vi "Grain Boundary Genie, 2014-07-30.vi"() -> ()   [LabVIEW 2010]
uses:
  <vilib>/Analysis/NI_AALBase.lvlib
  <vilib>/Analysis/baseanly.llb/Real Dot Product.vi
  <vilib>/Analysis/NI_AALPro.lvlib
  <vilib>/Analysis/_algsub.llb/Real Vector Norm.vi
  <vilib>/picture/3D Picture Control/NI_3D Picture Control.lvlib
  <vilib>/Analysis/baseanly.llb/A x Vector.vi
  <vilib>/Analysis/baseanly.llb/Vector x A.vi
  <vilib>/Analysis/baseanly.llb/Real A x B.vi
  <vilib>/Utility/file.llb/Write To Spreadsheet File (string).vi
panel:
  out "x/y":dbl[](array[numeric])
  out "Cross Product 2":dbl[](array[numeric])
  out "Cross Product":dbl[](array[numeric])
  out "Lattice Parameter":dbl=6.615785553057252
  in  "Make GB":bool=TRUE
  out "STEM Viewing Angles Array":dbl[][](array[numeric])=[[0.0, 1.0, 0.0], [0.0, 0.0, 1.0], [0.0, 1.0, 1.0], [0.0, -1.0, 1.0], [0.0, 1.0, -1.0]]
  in  "Make Grain 2":bool=TRUE
  in  "Make Grain 1":bool=TRUE
  out "Grain 2 Primative":T1={"Structure Name"="CdTe", "Lattice vector a"=[0.0, 0.0, 6.615785553057252], "Lattice vector b"=[6.615785553057252, 0.0, 0.0], "Lattice vector c"=[0.0, -6.615785553057252, 0.0], "Atoms Array"=[{"Atom Name"="Cd", "Positions (Direct)"=[[0.0, 0.0, 0.0], [0.0, 0.5, 0.5], [0.5, 0.0, 0.5], [0.5, 0.5, 0.0]], "Positions (Cartesian)"=[[0.0, 0.0, 0.0], [3.307892776528626, -3.307892776528626, 0.0], [0.0, -3.307892776528626, 3.307892776528626], [3.307892776528626, 0.0, 3.307892776528626]]}, {"Atom Name"="Te", "Positions (Direct)"=[[0.25, 0.25, 0.25], [0.75, 0.75, 0.25], [0.75, 0.25, 0.75], [0.25, 0.75, 0.75]], "Positions (Cartesian)"=[[1.653946388264313, -1.653946388264313, 1.653946388264313], [4.96183916479294, -1.653946388264313, 4.96183916479294], [1.653946388264313, -4.96183916479294, 4.96183916479294], [4.96183916479294, -4.96183916479294, 1.653946388264313]]}], "# of atoms"=8} {"Atoms Array"."Positions (Cartesian)" format="%#_4f"; "Atoms Array"."Positions (Direct)" format="%#_4f"}
  out "Grain 1 Primitive":T1={"Structure Name"="CdTe", "Lattice vector a"=[0.0, 0.0, 6.615785553057252], "Lattice vector b"=[6.615785553057252, 0.0, 0.0], "Lattice vector c"=[0.0, -6.615785553057252, 0.0], "Atoms Array"=[{"Atom Name"="Cd", "Positions (Direct)"=[[0.0, 0.0, 0.0], [0.0, 0.5, 0.5], [0.5, 0.0, 0.5], [0.5, 0.5, 0.0]], "Positions (Cartesian)"=[[0.0, 0.0, 0.0], [3.307892776528626, -3.307892776528626, 0.0], [0.0, -3.307892776528626, 3.307892776528626], [3.307892776528626, 0.0, 3.307892776528626]]}, {"Atom Name"="Te", "Positions (Direct)"=[[0.25, 0.25, 0.25], [0.75, 0.75, 0.25], [0.75, 0.25, 0.75], [0.25, 0.75, 0.75]], "Positions (Cartesian)"=[[1.653946388264313, -1.653946388264313, 1.653946388264313], [4.96183916479294, -1.653946388264313, 4.96183916479294], [1.653946388264313, -4.96183916479294, 4.96183916479294], [4.96183916479294, -4.96183916479294, 1.653946388264313]]}], "# of atoms"=8} {"Atoms Array"."Positions (Cartesian)" format="%#_4f"; "Atoms Array"."Positions (Direct)" format="%#_4f"}
  in  "Load GB VESTA":bool
  in  "Load G2 VESTA":bool
  in  "Load G1 VESTA":bool
  out "Viewable?":bool=TRUE
  in  "Grain 1 Start":dbl
  in  "Conventional Unit Cell":T1={"Structure Name"="CdTe", "Lattice vector a"=[6.615785553057252, 0.0, 0.0], "Lattice vector b"=[0.0, 6.615785553057252, 0.0], "Lattice vector c"=[0.0, 0.0, 6.615785553057252], "Atoms Array"=[{"Atom Name"="Cd", "Positions (Direct)"=[[0.0, 0.0, 0.0], [0.0, 0.5, 0.5], [0.5, 0.0, 0.5], [0.5, 0.5, 0.0]], "Positions (Cartesian)"=[[0.0, 0.0, 0.0], [0.0, 3.307892776528626, 3.307892776528626], [3.307892776528626, 0.0, 3.307892776528626], [3.307892776528626, 3.307892776528626, 0.0]]}, {"Atom Name"="Te", "Positions (Direct)"=[[0.25, 0.25, 0.25], [0.75, 0.75, 0.25], [0.75, 0.25, 0.75], [0.25, 0.75, 0.75]], "Positions (Cartesian)"=[[1.653946388264313, 1.653946388264313, 1.653946388264313], [4.96183916479294, 4.96183916479294, 1.653946388264313], [4.96183916479294, 1.653946388264313, 4.96183916479294], [1.653946388264313, 4.96183916479294, 4.96183916479294]]}], "# of atoms"=8}
  in  "Overlap Region":dbl(slide) scale=-2.0..2.0
  in  "Tab Control":T2(tab)=enum."Analysis"
  in  "Remove Close Atoms":bool
  out "Subset for Y?":bool
  out "Repeating Y Length Scale":dbl=99.01964045547014
  in  "Crop to Smallest Repeating":bool
  in  "Slab Y":dbl=6.0
  in  "Slab X":dbl=6.0
  out "Subset for X?":bool
  in  "Tolerance (A)":dbl=1.0
  in  "Presorted?":bool
  out "Repeating X Length Scale":dbl=99.01964045547014
  in  "Minimally Allowable Distance (A)":dbl=1.5
  out "# of Atoms Removed":i32
  in  "Options":cluster{"Border?":bool, "Bonds?":bool}={"Border?"=TRUE, "Bonds?"=FALSE}
  in  "Scale":dbl(slide)=0.06161137440758294 scale=0.0..0.2
  in  "Mutual Viewing Angle":dbl[](array[numeric])=[0.0, 1.0, 0.0]
  in  "STEM Viewing Angles":u16(ring) items=["[0,0,1]", "[1,-1,0]", "[-1,1,0]"]
  out "# of Atoms":i32=36
  out "Atoms / A³":dbl=0.06216246776245014
  out "% of Bulk atomic density":dbl=2.250005167366452
  out "Grain 2 Integers":dbl[](array[numeric])=[1.0, 0.0, 0.0]
  out "Grain 1 Integers":dbl[](array[numeric])=[1.0, 0.0, 0.0]
  out "Misorientation Angle":dbl
  out "Suggested Viewing Angle":dbl[](array[numeric])=[0.0, 1.0, 0.0]
  in  "Suggest Sizes":bool
  in  "Tolerance":dbl=0.01
  in  "Grain 2 Max Length (A)":dbl=10.0
  in  "Grain 1 Max Length (A)":dbl=10.0
  in  "Max Grain Width":dbl=1.0
  in  "Grain 2 Min Length":dbl=1.0
  in  "Grain 1 Min Length (A)":dbl=1.0
  in  "Max Grain Height":dbl=1.0
  in  "Structure Name":string="(0.0) twist [1,0,0] [1,0,0+0.0tilt] (0.00,0.00,0.00)T GB"
  in  "Save to POSCAR":bool
  in  "Relaxation Type":string(combo)="conv opti"
  in  "Make into GULP":bool
  out "Grain Boundary Object":refnum<vi>
  out "Grain 2 Object":refnum<vi>
  out "Grain 1 Object":refnum<vi>
  in  "Add Tilt Angle":dbl(slide) scale=0.0..90.0
  out "Grain Boundary":T1={"Structure Name"="(0.0) twist [1,0,0] [1,0,0+0.0tilt] (0.00,0.00,0.00)T GB", "Lattice vector a"=[6.615785553057252, 0.0, 0.0], "Lattice vector b"=[0.0, 6.615785553057252, 0.0], "Lattice vector c"=[0.0, 0.0, 13.231571106114504], "Atoms Array"=[{"Atom Name"="Cd", "Positions (Direct)"=[[0.0, 0.0, 0.0], [0.0, 0.0, 0.5], [0.0, 0.5, 0.25], [0.0, 1.0, 0.0], [0.0, 1.0, 0.5], [0.5, 0.0, 0.25], [0.5, 0.5, 0.0], [0.5, 0.5, 0.5], [0.5, 1.0, 0.25], [1.0, 0.0, 0.0], [1.0, 0.0, 0.5], [1.0, 0.5, 0.25], [1.0, 1.0, 0.0], [1.0, 1.0, 0.5], [0.0, 0.0, 0.5], [0.0, 0.0, 1.0], [0.0, 0.5, 0.75], [0.0, 1.0, 0.5], [0.0, 1.0, 1.0], [0.5, 0.0, 0.75], [0.5, 0.5, 0.5], [0.5, 0.5, 1.0], [0.5, 1.0, 0.75], [1.0, 0.0, 0.5], [1.0, 0.0, 1.0], [1.0, 0.5, 0.75], [1.0, 1.0, 0.5], [1.0, 1.0, 1.0]], "Positions (Cartesian)"=[[0.0, 0.0, 0.0], [0.0, 0.0, 6.615785553057252], [0.0, 3.307892776528626, 3.307892776528626], [0.0, 6.615785553057252, 0.0], [0.0, 6.615785553057252, 6.615785553057252], [3.307892776528626, 0.0, 3.307892776528626], [3.307892776528626, 3.307892776528626, 0.0], [3.307892776528626, 3.307892776528626, 6.615785553057252], [3.307892776528626, 6.615785553057252, 3.307892776528626], [6.615785553057252, 0.0, 0.0], [6.615785553057252, 0.0, 6.615785553057252], [6.615785553057252, 3.307892776528626, 3.307892776528626], [6.615785553057252, 6.615785553057252, 0.0], [6.615785553057252, 6.615785553057252, 6.615785553057252], [0.0, 0.0, 6.615785553057252], [0.0, 0.0, 13.231571106114504], [0.0, 3.307892776528626, 9.92367832958588], [0.0, 6.615785553057252, 6.615785553057252], [0.0, 6.615785553057252, 13.231571106114504], [3.307892776528626, 0.0, 9.92367832958588], [3.307892776528626, 3.307892776528626, 6.615785553057252], [3.307892776528626, 3.307892776528626, 13.231571106114504], [3.307892776528626, 6.615785553057252, 9.92367832958588], [6.615785553057252, 0.0, 6.615785553057252], [6.615785553057252, 0.0, 13.231571106114504], [6.615785553057252, 3.307892776528626, 9.92367832958588], [6.615785553057252, 6.615785553057252, 6.615785553057252], [6.615785553057252, 6.615785553057252, 13.231571106114504]]}, {"Atom Name"="Te", "Positions (Direct)"=[[0.25, 0.24999999999999992, 0.375], [0.25, 0.75, 0.125], [0.75, 0.24999999999999992, 0.125], [0.75, 0.75, 0.375], [0.25, 0.24999999999999992, 0.875], [0.25, 0.75, 0.625], [0.75, 0.24999999999999992, 0.625], [0.75, 0.75, 0.875]], "Positions (Cartesian)"=[[1.653946388264313, 1.6539463882643126, 4.96183916479294], [1.653946388264313, 4.96183916479294, 1.653946388264313], [4.96183916479294, 1.6539463882643126, 1.653946388264313], [4.96183916479294, 4.96183916479294, 4.96183916479294], [1.653946388264313, 1.6539463882643126, 11.577624717850192], [1.653946388264313, 4.96183916479294, 8.269731941321565], [4.96183916479294, 1.6539463882643126, 8.269731941321565], [4.96183916479294, 4.96183916479294, 11.577624717850192]]}], "# of atoms"=36} {"Atoms Array"."Positions (Cartesian)" format="%#_4f"; "Atoms Array"."Positions (Direct)" format="%#_4f"}
  out "Grain 2":T1={"Structure Name"="CdTe Expanded to Box", "Lattice vector a"=[6.615785553057252, 0.0, 0.0], "Lattice vector b"=[0.0, 6.615785553057252, 0.0], "Lattice vector c"=[0.0, 0.0, 6.615785553057252], "Atoms Array"=[{"Atom Name"="Cd", "Positions (Direct)"=[[0.0, 0.0, 0.0], [0.0, 0.0, 1.0], [0.0, 0.5, 0.5], [0.0, 1.0, 0.0], [0.0, 1.0, 1.0], [0.5, 0.0, 0.5], [0.5, 0.5, 0.0], [0.5, 0.5, 1.0], [0.5, 1.0, 0.5], [1.0, 0.0, 0.0], [1.0, 0.0, 1.0], [1.0, 0.5, 0.5], [1.0, 1.0, 0.0], [1.0, 1.0, 1.0]], "Positions (Cartesian)"=[[0.0, 0.0, 0.0], [0.0, 0.0, 6.615785553057252], [0.0, 3.307892776528626, 3.307892776528626], [0.0, 6.615785553057252, 0.0], [0.0, 6.615785553057252, 6.615785553057252], [3.307892776528626, 0.0, 3.307892776528626], [3.307892776528626, 3.307892776528626, 0.0], [3.307892776528626, 3.307892776528626, 6.615785553057252], [3.307892776528626, 6.615785553057252, 3.307892776528626], [6.615785553057252, 0.0, 0.0], [6.615785553057252, 0.0, 6.615785553057252], [6.615785553057252, 3.307892776528626, 3.307892776528626], [6.615785553057252, 6.615785553057252, 0.0], [6.615785553057252, 6.615785553057252, 6.615785553057252]]}, {"Atom Name"="Te", "Positions (Direct)"=[[0.25, 0.24999999999999992, 0.75], [0.25, 0.75, 0.25], [0.75, 0.24999999999999992, 0.25], [0.75, 0.75, 0.75]], "Positions (Cartesian)"=[[1.653946388264313, 1.6539463882643126, 4.96183916479294], [1.653946388264313, 4.96183916479294, 1.653946388264313], [4.96183916479294, 1.6539463882643126, 1.653946388264313], [4.96183916479294, 4.96183916479294, 4.96183916479294]]}], "# of atoms"=18} {"Atoms Array"."Positions (Cartesian)" format="%#_4f"; "Atoms Array"."Positions (Direct)" format="%#_4f"}
  out "Grain 1":T1={"Structure Name"="CdTe Expanded to Box", "Lattice vector a"=[6.681943408587824, 0.0, 0.0], "Lattice vector b"=[0.0, 6.681943408587824, 0.0], "Lattice vector c"=[0.0, 0.0, 6.615785553057252], "Atoms Array"=[{"Atom Name"="Cd", "Positions (Direct)"=[[0.0, 0.0, 0.0], [0.0, 0.0, 1.0], [0.0, 0.49504950495049505, 0.5], [0.0, 0.9900990099009901, 0.0], [0.0, 0.9900990099009901, 1.0], [0.49504950495049505, 0.0, 0.5], [0.49504950495049505, 0.49504950495049505, 0.0], [0.49504950495049505, 0.49504950495049505, 1.0], [0.49504950495049505, 0.9900990099009901, 0.5], [0.9900990099009901, 0.0, 0.0], [0.9900990099009901, 0.0, 1.0], [0.9900990099009901, 0.49504950495049505, 0.5], [0.9900990099009901, 0.9900990099009901, 0.0], [0.9900990099009901, 0.9900990099009901, 1.0]], "Positions (Cartesian)"=[[0.0, 0.0, 0.0], [0.0, 0.0, 6.615785553057252], [0.0, 3.307892776528626, 3.307892776528626], [0.0, 6.615785553057252, 0.0], [0.0, 6.615785553057252, 6.615785553057252], [3.307892776528626, 0.0, 3.307892776528626], [3.307892776528626, 3.307892776528626, 0.0], [3.307892776528626, 3.307892776528626, 6.615785553057252], [3.307892776528626, 6.615785553057252, 3.307892776528626], [6.615785553057252, 0.0, 0.0], [6.615785553057252, 0.0, 6.615785553057252], [6.615785553057252, 3.307892776528626, 3.307892776528626], [6.615785553057252, 6.615785553057252, 0.0], [6.615785553057252, 6.615785553057252, 6.615785553057252]]}, {"Atom Name"="Te", "Positions (Direct)"=[[0.24752475247524752, 0.24752475247524747, 0.75], [0.24752475247524752, 0.7425742574257427, 0.25], [0.7425742574257427, 0.24752475247524747, 0.25], [0.7425742574257427, 0.7425742574257427, 0.75]], "Positions (Cartesian)"=[[1.653946388264313, 1.6539463882643126, 4.96183916479294], [1.653946388264313, 4.96183916479294, 1.653946388264313], [4.96183916479294, 1.6539463882643126, 1.653946388264313], [4.96183916479294, 4.96183916479294, 4.96183916479294]]}], "# of atoms"=18} {"Atoms Array"."Positions (Cartesian)" format="%#_4f"; "Atoms Array"."Positions (Direct)" format="%#_4f"}
  in  "Primitive Lattice Vectors":T1={"Structure Name"="Relax2 Subcrystal", "Lattice vector a"=[0.0, 3.3046962263585, 3.3046962263585], "Lattice vector b"=[3.3046962263585, 0.0, 3.3046962263585], "Lattice vector c"=[3.3046962263585, 3.3046962263585, 0.0], "Atoms Array"=[{"Atom Name"="Cd", "Positions (Direct)"=[[0.0, 0.0, 0.0]], "Positions (Cartesian)"=[[0.0, 0.0, 0.0]]}, {"Atom Name"="Te", "Positions (Direct)"=[[0.25, 0.25, 0.25]], "Positions (Cartesian)"=[[1.65234811317925, 1.65234811317925, 1.65234811317925]]}], "# of atoms"=2} {"Atoms Array"."Positions (Cartesian)" format="%#_4f"; "Atoms Array"."Positions (Direct)" format="%#_4f"}
  out "Grain Boundary Render":refnum<vi>(3d-picture)
  in  "Translation Vector":dbl[](array[slide])=[0.0, 0.0, 0.0] scale=0.0..2.0
  in  "Twist Angle":dbl(slide) scale=0.0..90.0
  in  "Grain 2 Orientation":dbl[](array[numeric])=[1.0, 0.0, 0.0]
  in  "Grain 1 Orientation":dbl[](array[numeric])=[1.0, 0.0, 0.0]
  out "Grain 2 Render":refnum<vi>(3d-picture)
  out "Grain 1 Render":refnum<vi>(3d-picture)
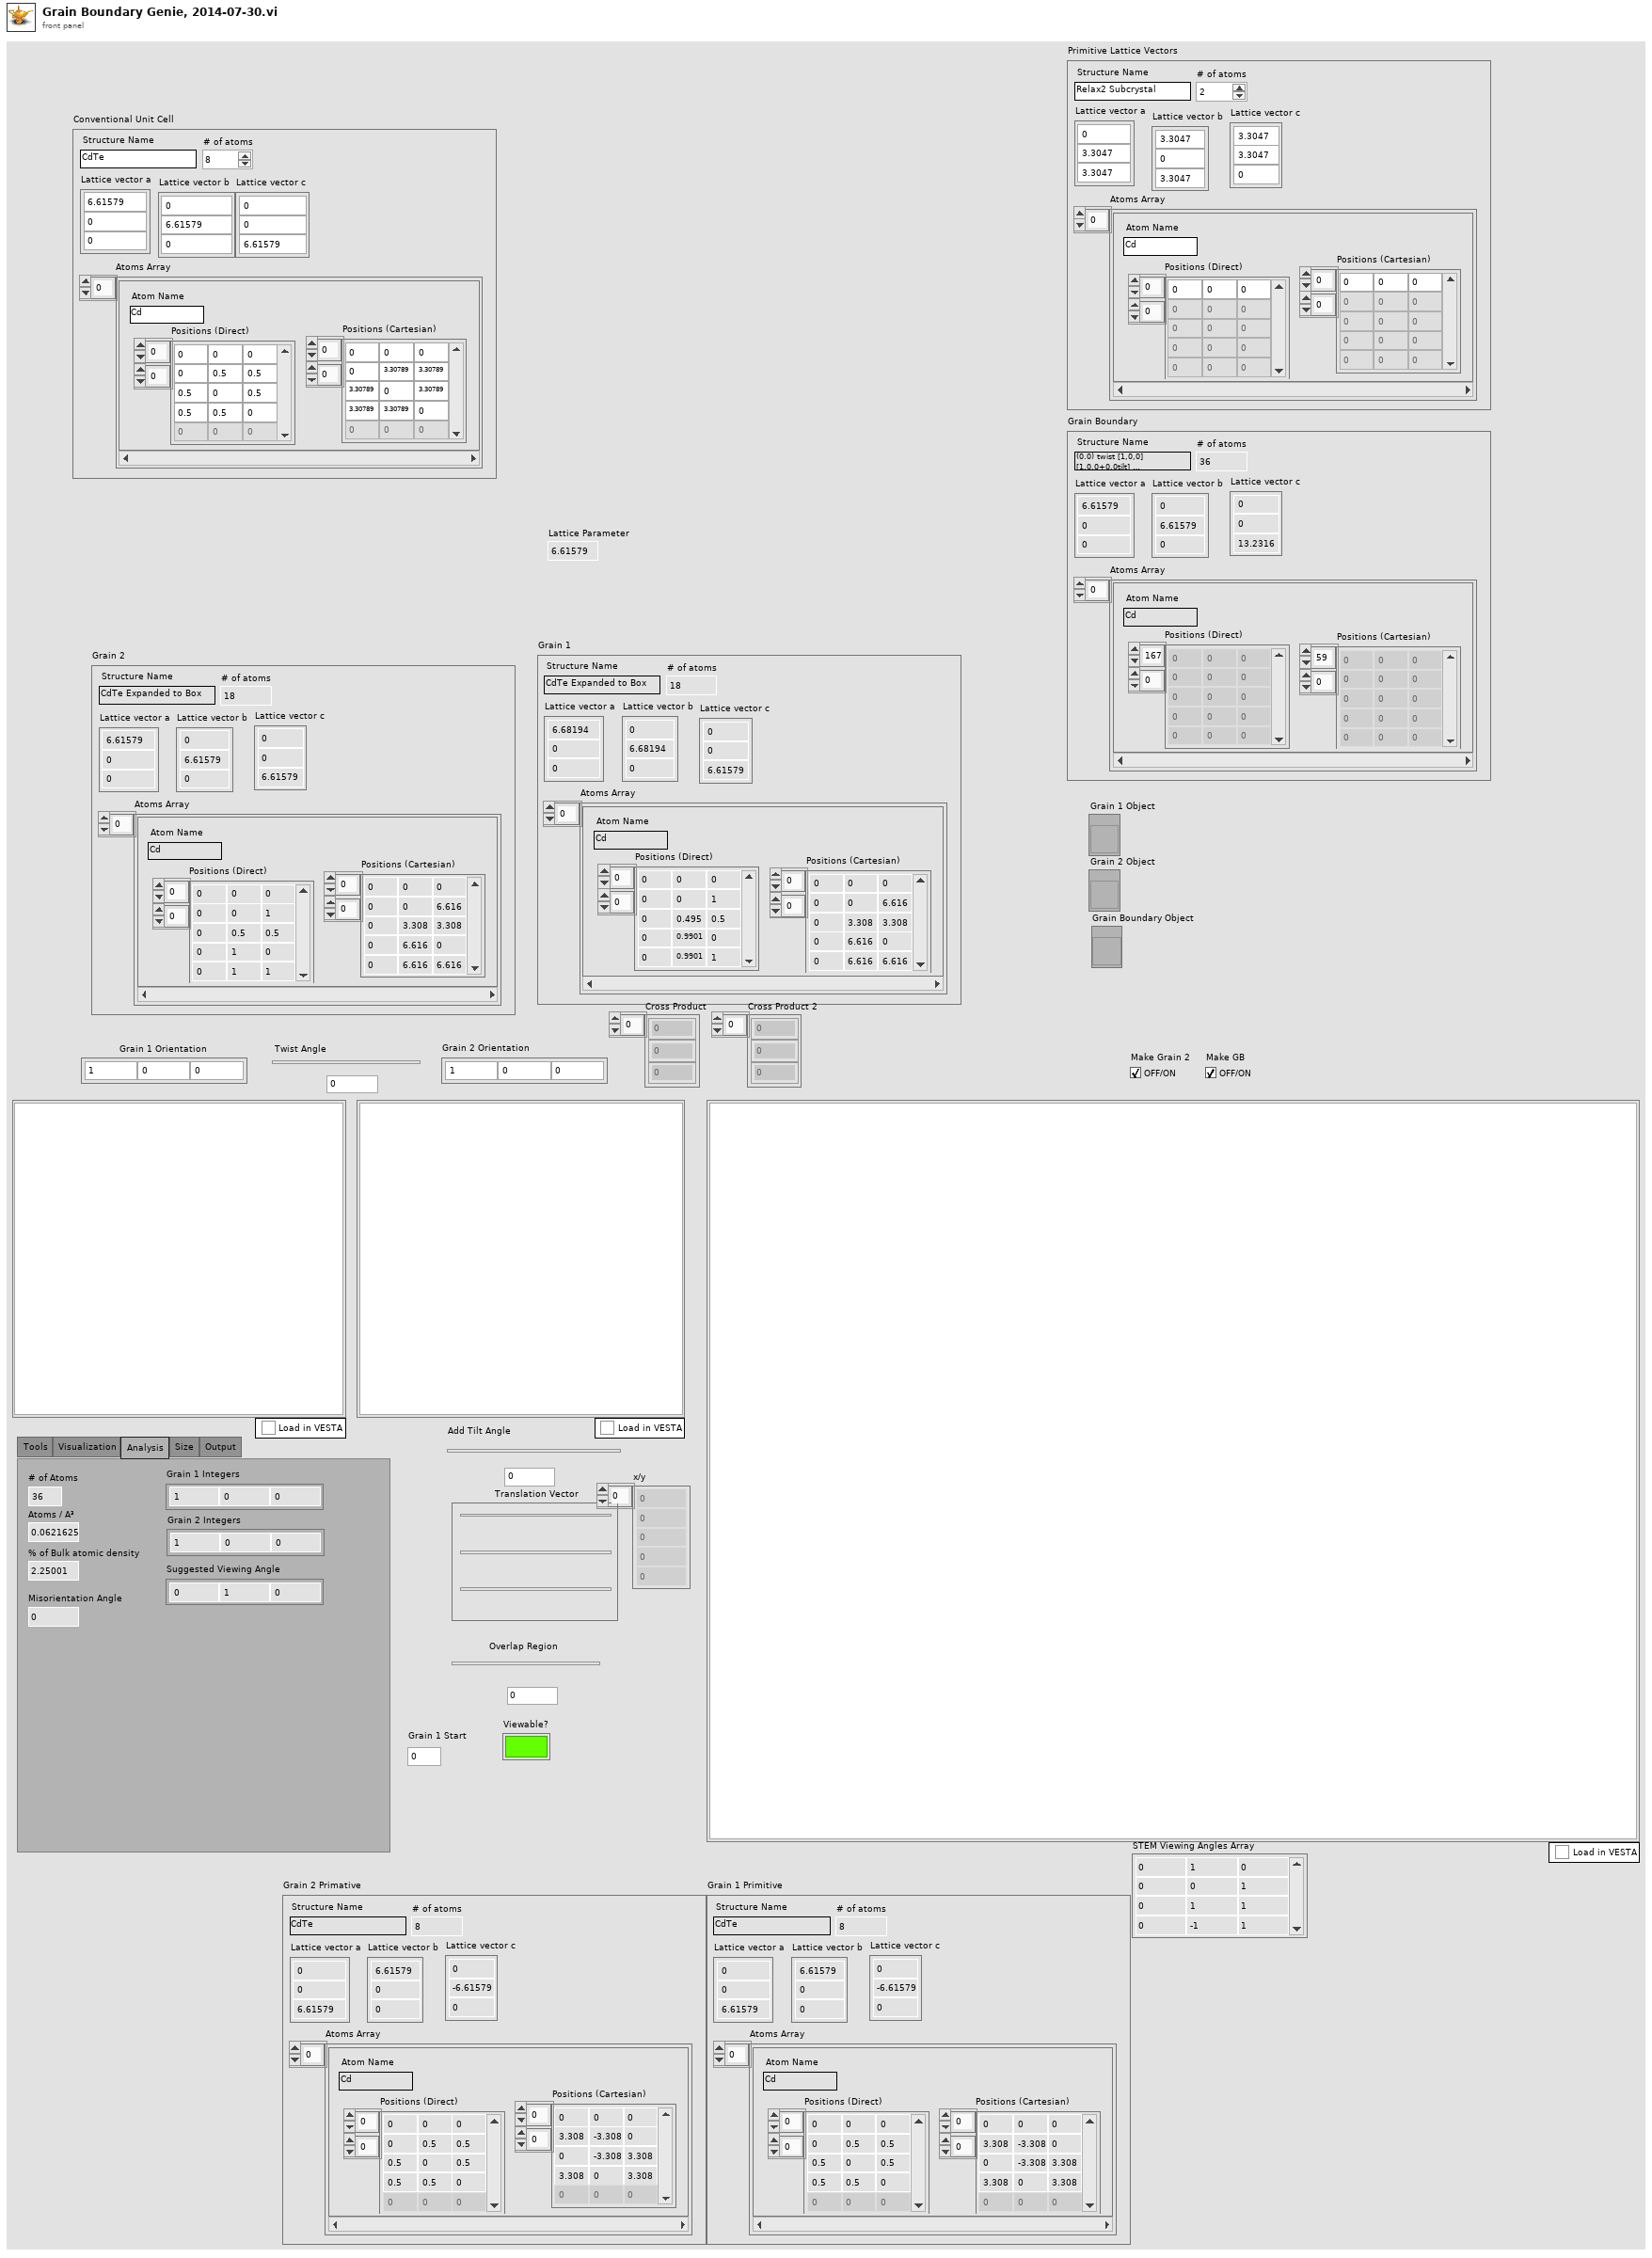
[diagram p1: front panel]
types:
  T1 = cluster{"Structure Name":string, "Lattice vector a":dbl[], "Lattice vector b":dbl[], "Lattice vector c":dbl[], "Atoms Array":cluster{"Atom Name":string, "Positions (Direct)":dbl[][], "Positions (Cartesian)":dbl[][]}[], "# of atoms":i32}
  T2 = enum32{"Tools", "Visualization", "Analysis", "Size", "Output"}
  T3 = typedef "NI_Matrix.lvlib/RealMatrix.ctl" = dbl[][]
  T4 = cluster{"Z Min":dbl, "Max Grain Width":dbl, "Z Min":dbl, "Max Grain Height":dbl, "Grain 1 Start":dbl, "Grain 1 Min Length (A)":dbl}
  T5 = cluster{"Grain 1 Start":dbl, "Max Grain Width":dbl, "Grain 1 Start":dbl, "Max Grain Height":dbl, dbl, "Grain 2 Min Length":dbl}
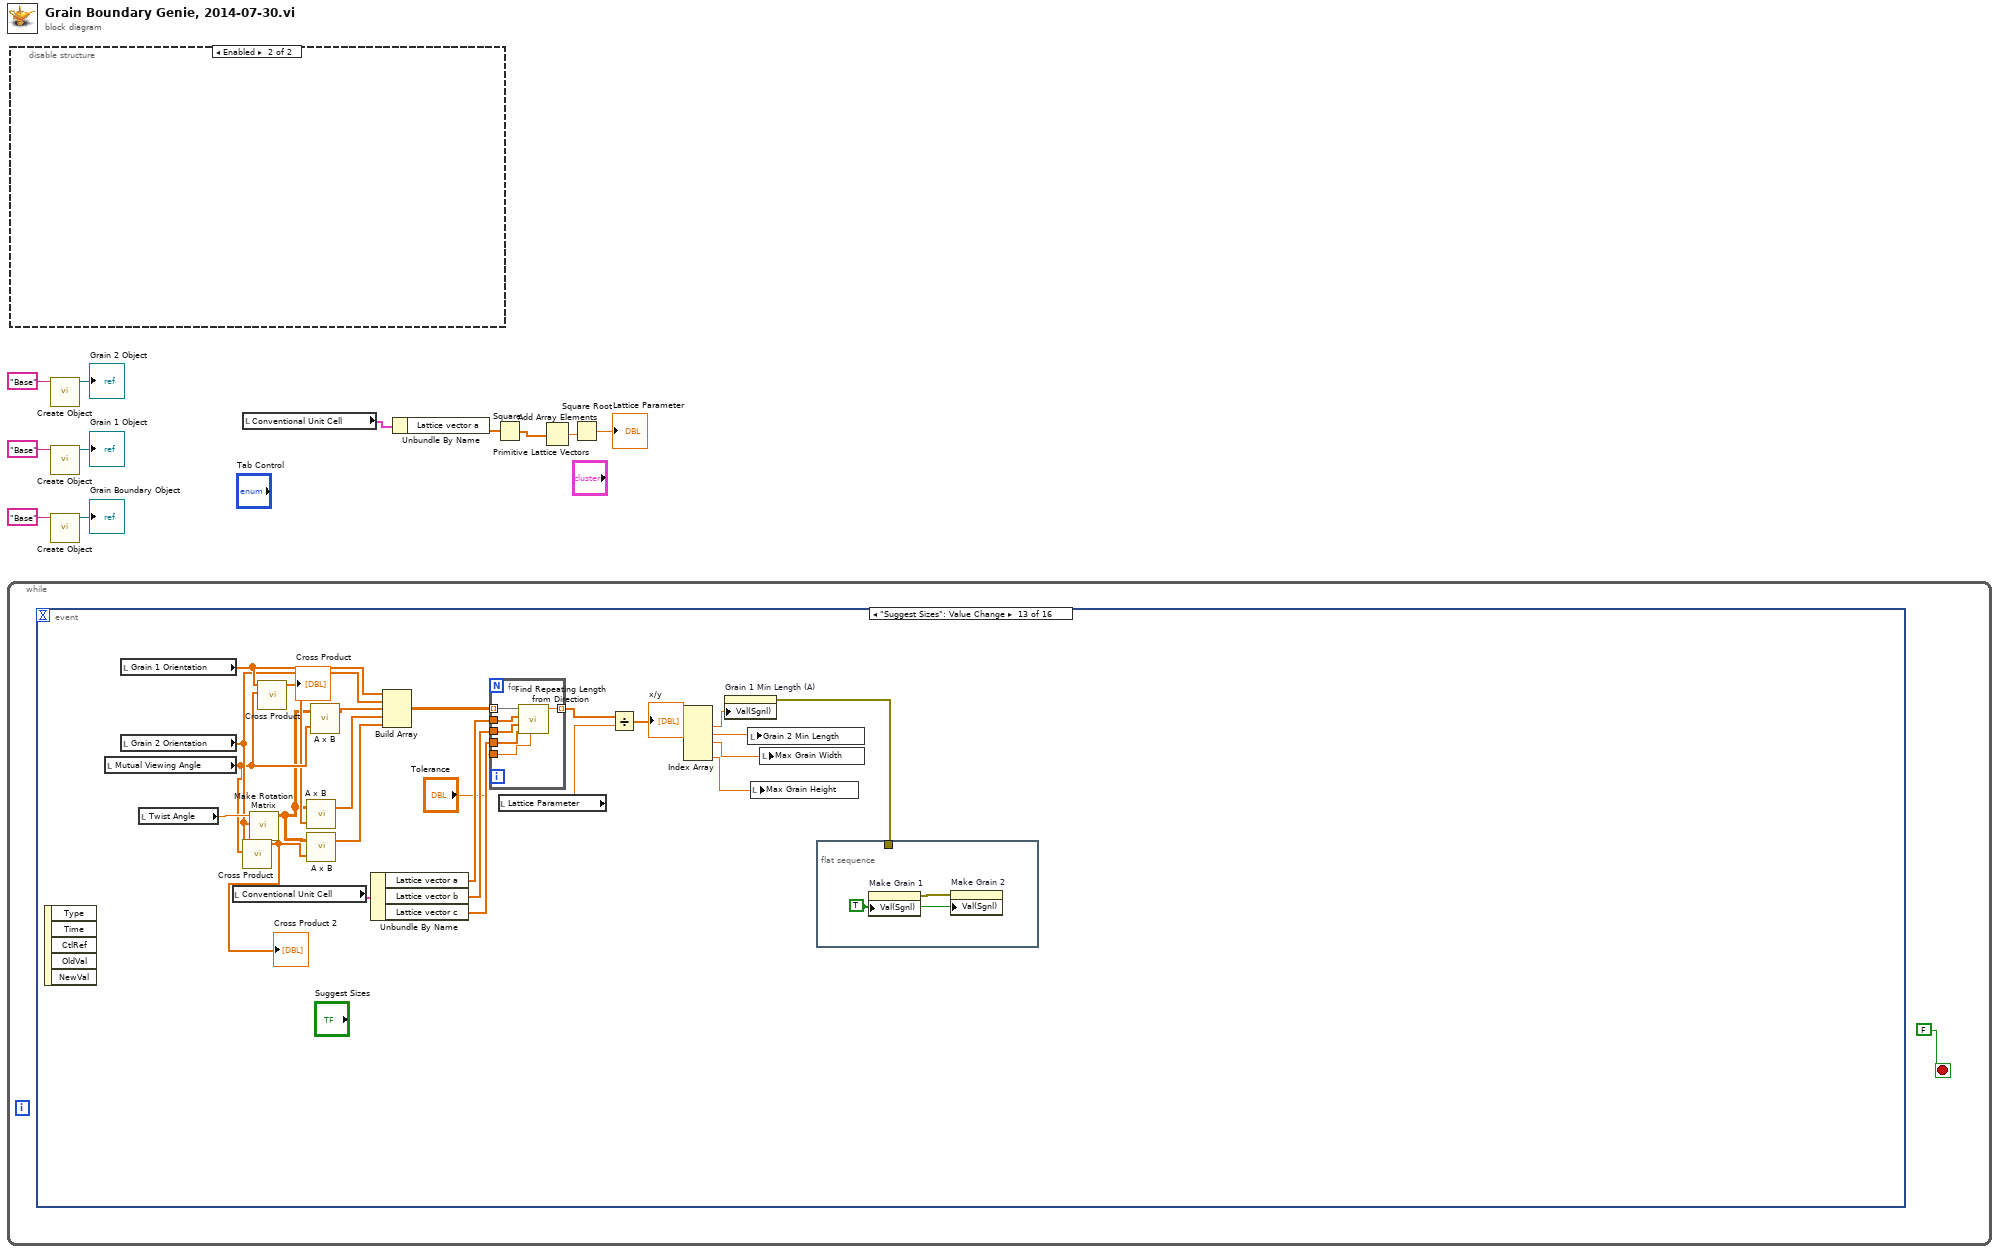
[diagram p0: block diagram]
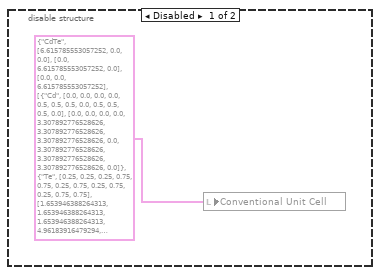
[diagram p2: hidden frame]
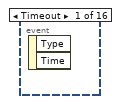
[diagram p3: hidden frame]
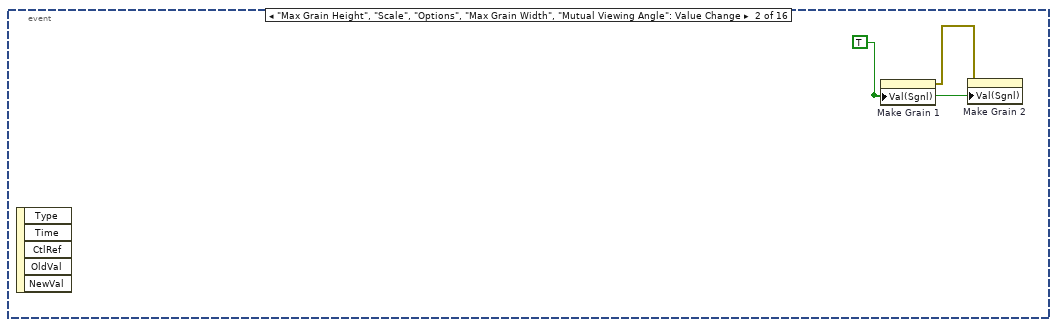
[diagram p4: hidden frame]
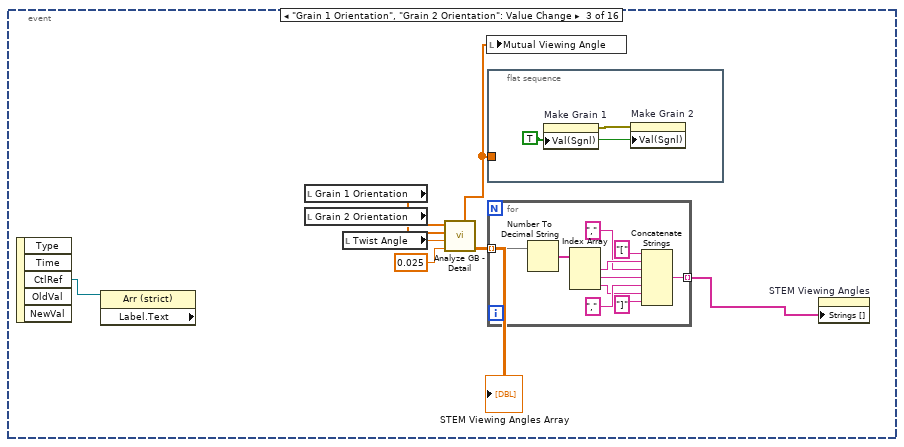
[diagram p5: hidden frame]
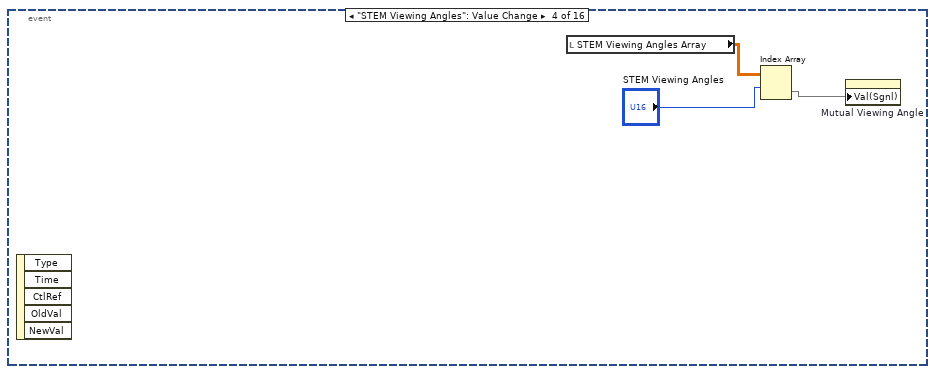
[diagram p6: hidden frame]
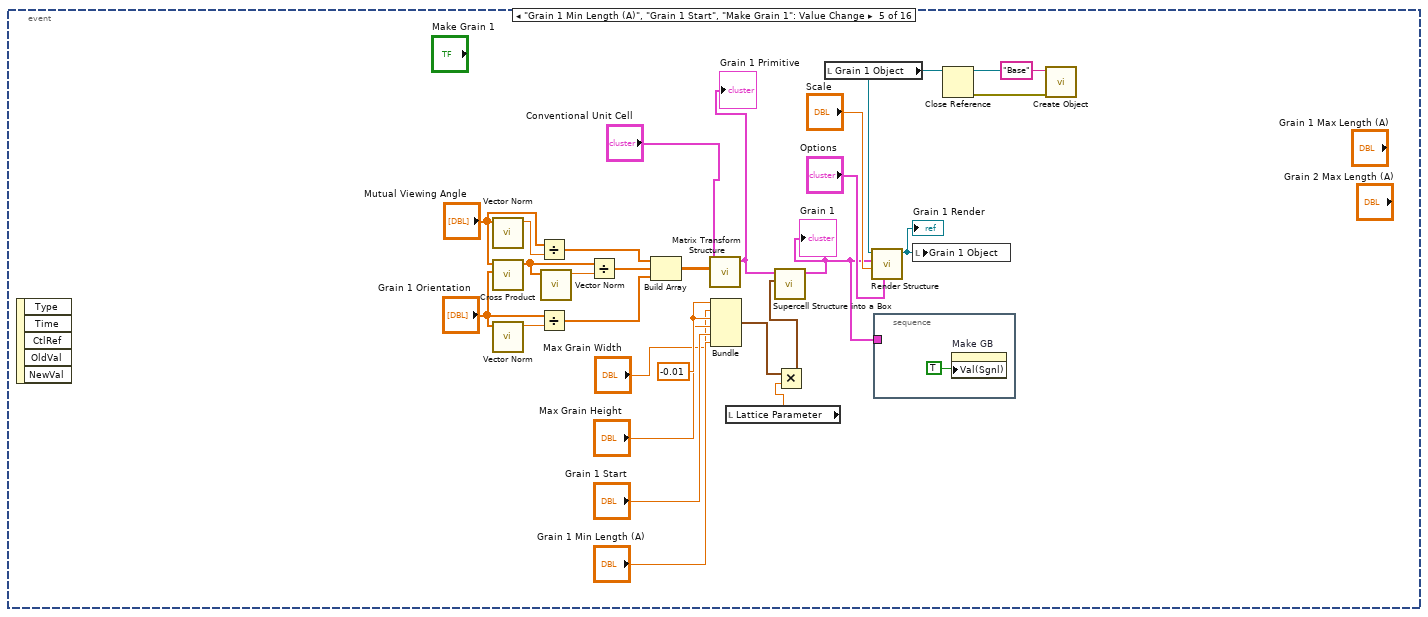
[diagram p7: hidden frame]
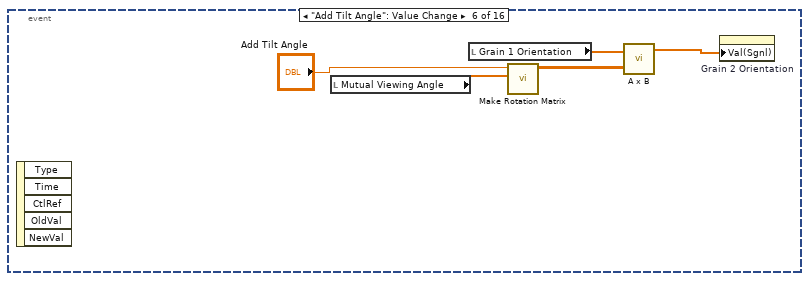
[diagram p8: hidden frame]
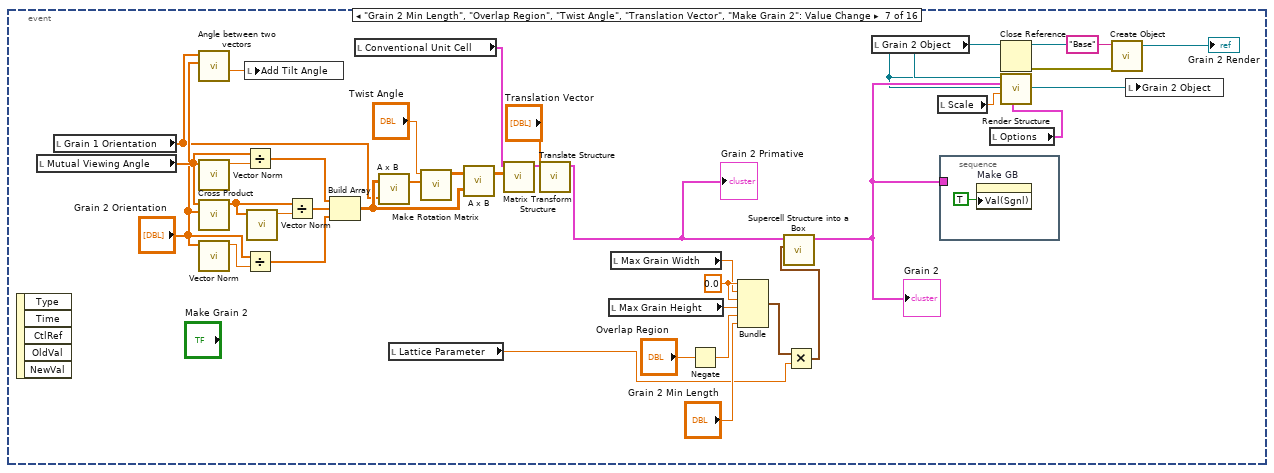
[diagram p9: hidden frame]
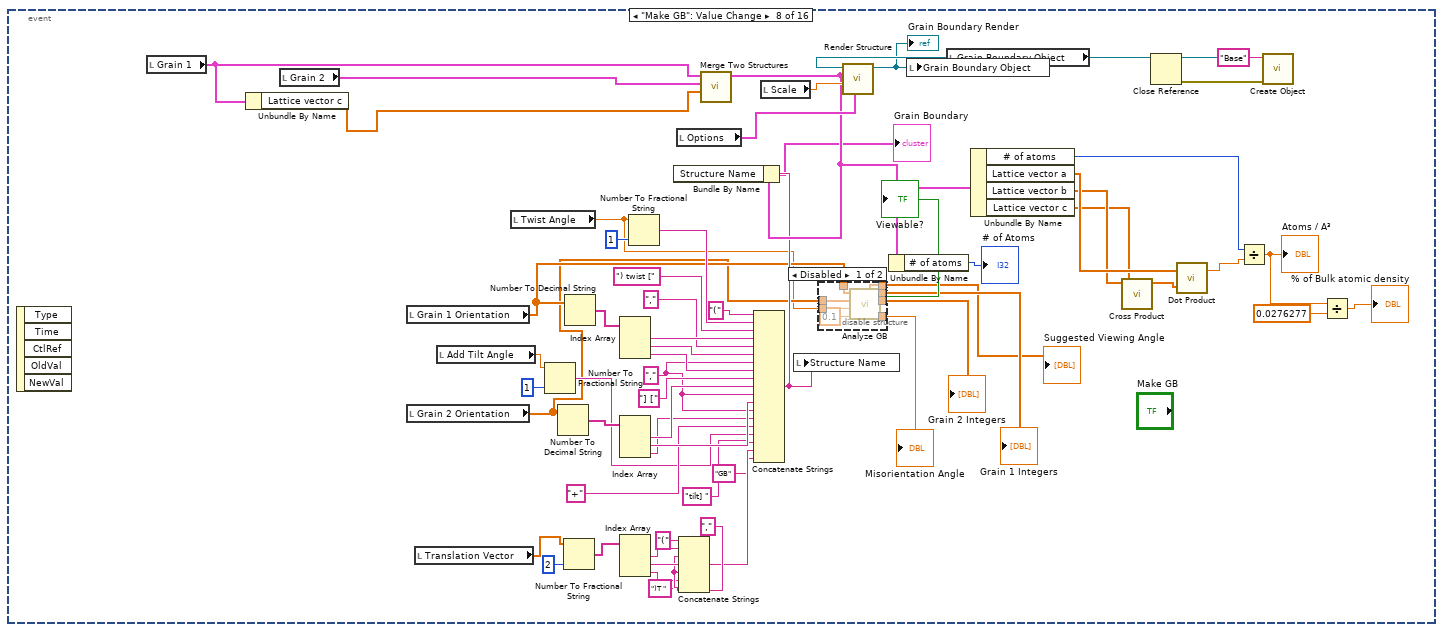
[diagram p10: hidden frame]
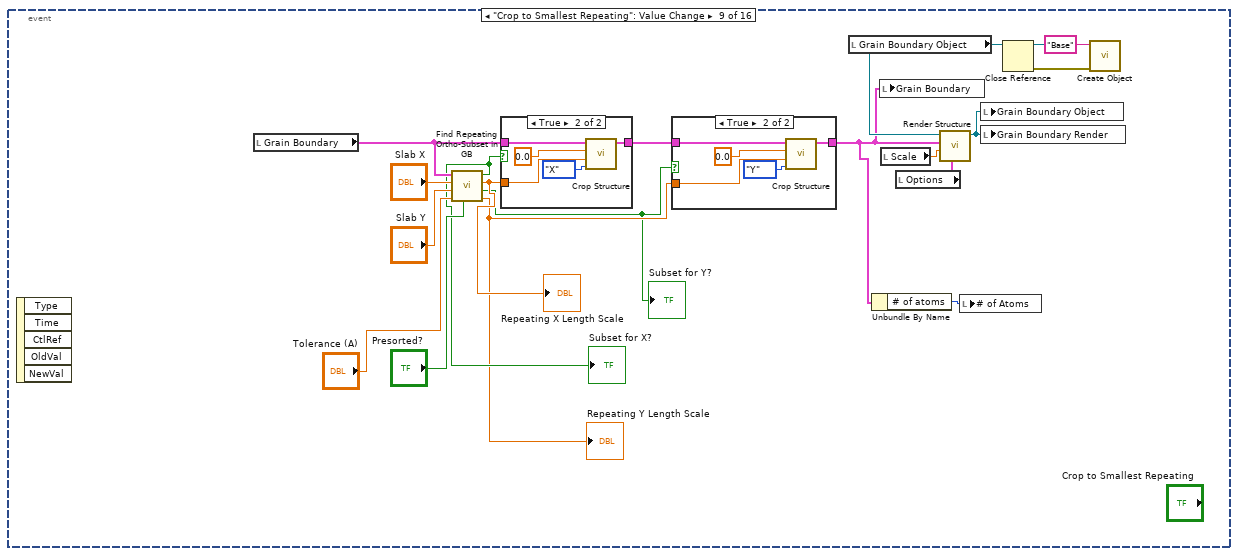
[diagram p12: hidden frame]
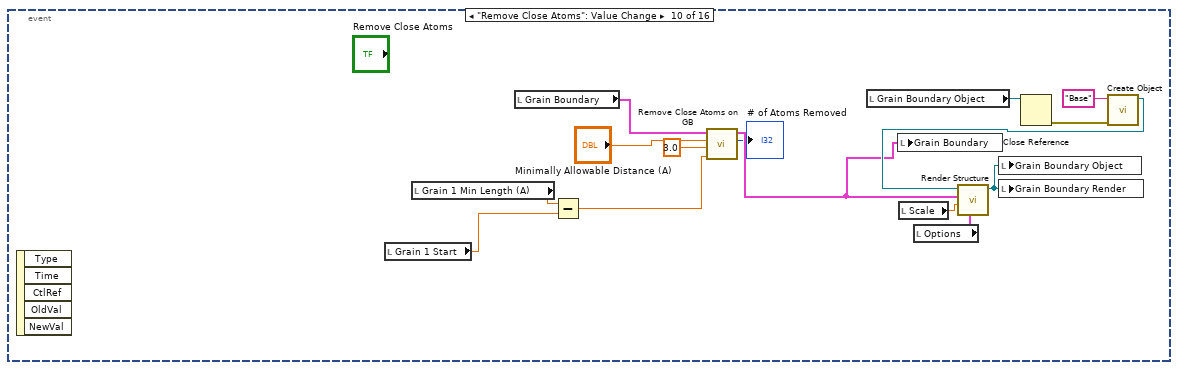
[diagram p15: hidden frame]
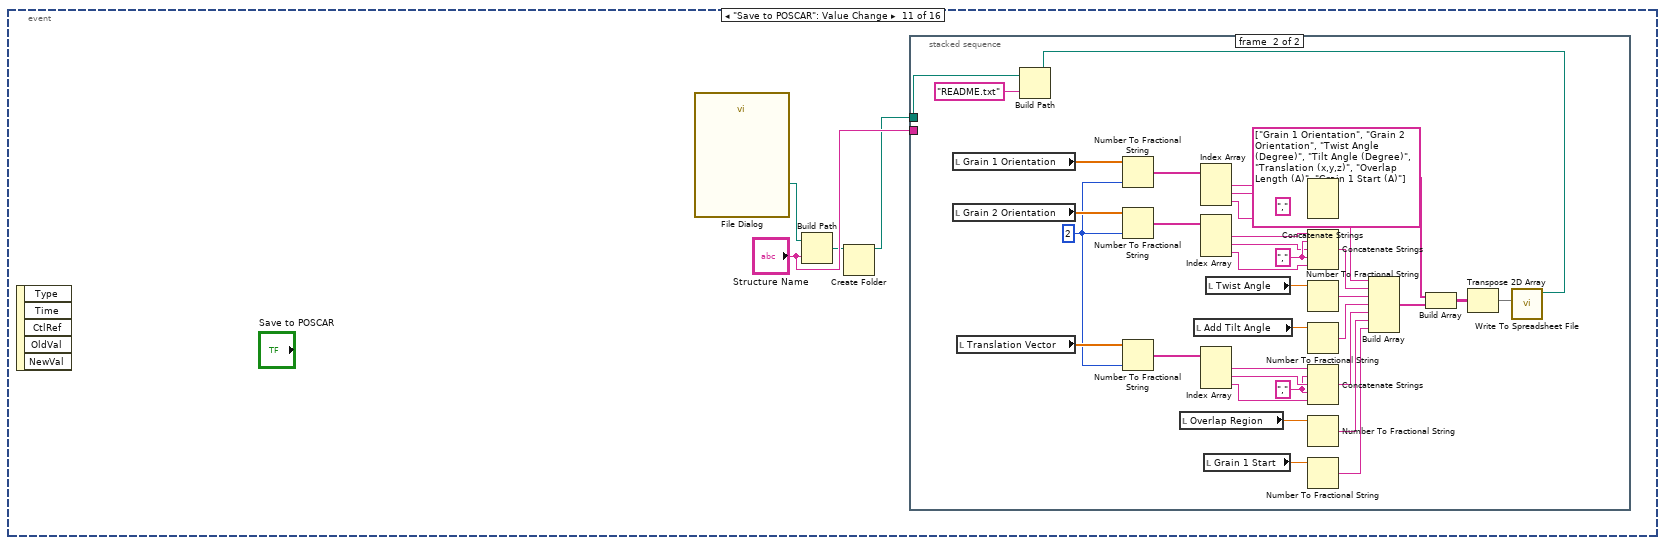
[diagram p16: hidden frame]
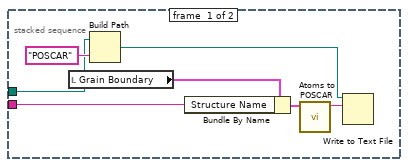
[diagram p17: hidden frame]
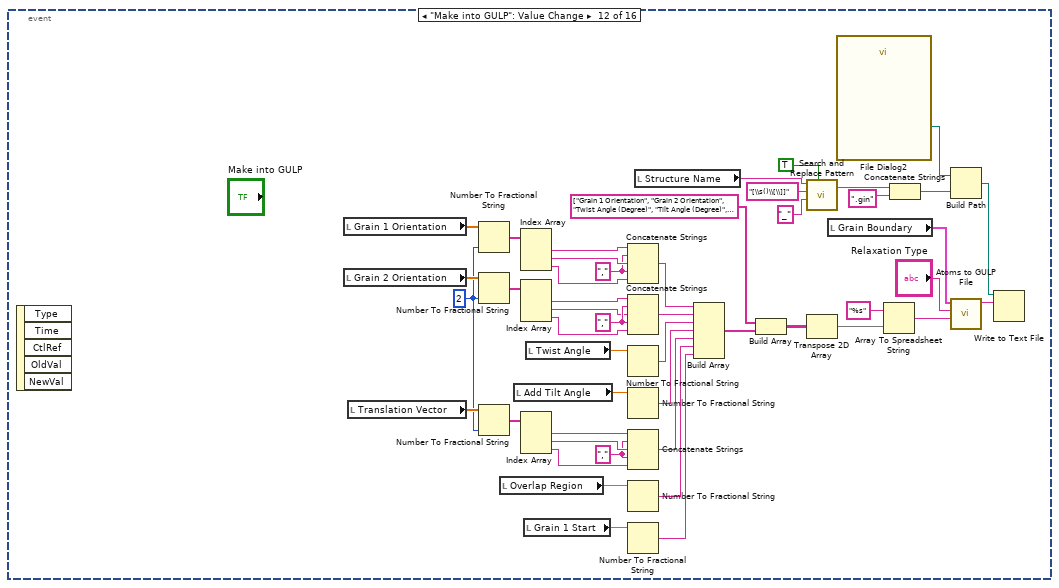
[diagram p18: hidden frame]
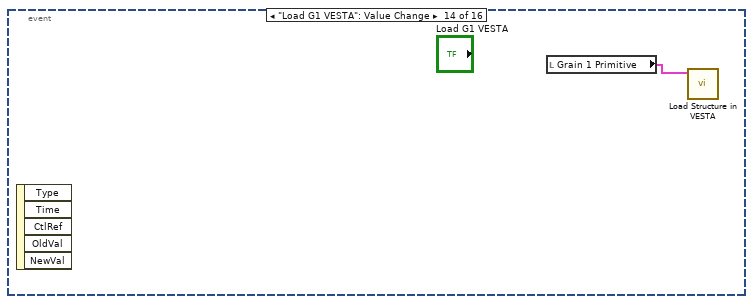
[diagram p19: hidden frame]
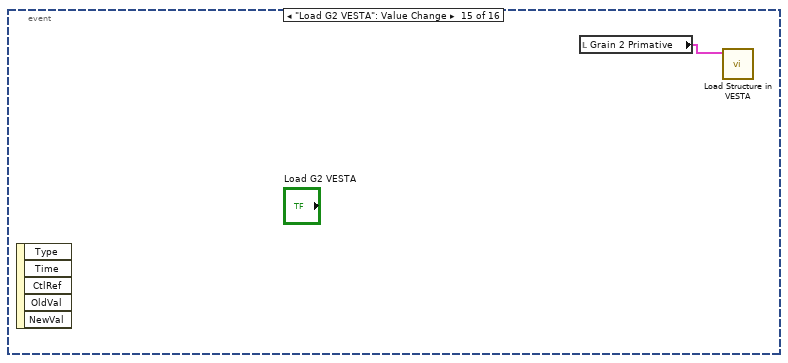
[diagram p20: hidden frame]
diagram:
  n1 = while {
    stop <- FALSE stop-if-true
    n2 = event shown="[12] \"Suggest Sizes\": Value Change" {
      selector: _ -> [_ _ _ _ _ _ _ _ _ _ _ _ _ _ _ _]
      dyn-events: _ -> [_ _ _ _ _ _ _ _ _ _ _ _ _ _ _ _]
      timeout: _ -> [_ _ _ _ _ _ _ _ _ _ _ _ _ _ _ _]
      event Timeout {
        n3 = event-data() -> ()  [unwired: 1 in, 2 out]
      }
      event "Max Grain Height", "Scale", "Options", "Max Grain Width", "Mutual Viewing Angle": Value Change {
        w14 = TRUE ("Value (Signaling)")
        n4 = event-data() -> ()  [unwired: 1 in, 5 out]
        n5 = property on="Make Grain 1" class="Bool (strict)"("Val(Sgnl)"=w14) -> (error out=w13:errorcluster)  [unwired: 2 in, 1 out]
        n6 = property on="Make Grain 2" class="Bool (strict)"(error in=w13, "Val(Sgnl)"=w14) -> ()  [unwired: 1 in, 2 out]
      }
      event "Grain 1 Orientation", "Grain 2 Orientation": Value Change {
        n7 = event-data() -> ("CtlRef"=w22:refnum<vi>)  [unwired: 1 in, 4 out]
        n8 = property class="Arr (strict)" props=["Label", "Text"](reference=w22) -> ()  [unwired: 1 in, 3 out]
        n9 = local read "Grain 1 Orientation"() -> (w21:dbl[])
        n10 = local read "Grain 2 Orientation"() -> (w20:dbl[])
        n11 = local read "Twist Angle"() -> (w19:dbl)
        n12 = call "Analyze GB - Detail.vi"("Integer Tolerance"=0.025, 9:w19, "Find Integer Rep?"=w20, "Grain Boundary Definition"=w21) -> ("STEM Viewing Angles"=w16:dbl[][], "Suggested view direction"=w17:dbl[])  [unwired: 6 out]
        "STEM Viewing Angles Array" <- w16
        n13 = local write "Mutual Viewing Angle"(w17) -> ()
        n14 = flat-sequence {
          tunnel: w17 -> [_]
          frame #0 {
            w34 = TRUE ("Value (Signaling)")
            n15 = property on="Make Grain 1" class="Bool (strict)"("Val(Sgnl)"=w34) -> (error out=w33:errorcluster)  [unwired: 2 in, 1 out]
            n16 = property on="Make Grain 2" class="Bool (strict)"(error in=w33, "Val(Sgnl)"=w34) -> ()  [unwired: 1 in, 2 out]
          }
        }
        n17 = for {
          tunnel: w16 -> [w32] mode=indexing
          tunnel: [w23] -> w15 mode=indexing
          n18 = Number To Decimal String(number=w32) -> (decimal integer string=w31:string[])  [unwired: 1 in]
          n19 = Index Array(array=w31) -> (element #1=w29:string, element #2=w27:string, element #3=w25:string)  [unwired: 3 in]
          n20 = Concatenate Strings("[" ("string"), w29, "," ("string"), w27, "," ("string"), w25, "]" ("string")) -> (w23:string)
        }
        n21 = property on="STEM Viewing Angles" class="Ring (strict)"("Strings []"=w15) -> ()  [unwired: 2 in, 2 out]
      }
      event "STEM Viewing Angles": Value Change {
        n22 = event-data() -> ()  [unwired: 1 in, 5 out]
        n23 = local read "STEM Viewing Angles Array"() -> (w37:dbl[][])
        n24 = Index Array(array=w37, index (row)="STEM Viewing Angles") -> (element=w35:dbl[])  [unwired: 1 in]
        n25 = property on="Mutual Viewing Angle" class="Arr (strict)"("Val(Sgnl)"=w35) -> ()  [unwired: 2 in, 2 out]
      }
      event "Grain 1 Min Length (A)", "Grain 1 Start", "Make Grain 1": Value Change {
        w59 = -0.01 ("Z Min")
        n26 = event-data() -> ()  [unwired: 1 in, 5 out]
        n27 = call-poly <vilib>:"Vector Norm.vi"("Input Vector"="Mutual Viewing Angle") -> ("norm"=w65:dbl)  [unwired: 9 in, 1 out]
        n28 = call <vilib>:"Cross Product.vi"("B Vector"="Grain 1 Orientation", "A Vector"="Mutual Viewing Angle") -> ("Cross Product"=w49:dbl[])  [unwired: 8 in, 1 out]
        n29 = call-poly <vilib>:"Vector Norm.vi"("Input Vector"="Grain 1 Orientation") -> ("norm"=w63:dbl)  [unwired: 9 in, 1 out]
        n30 = Divide(x="Mutual Viewing Angle", y=w65) -> (x/y=w62:dbl[])
        n31 = Divide(x="Grain 1 Orientation", y=w63) -> (x/y=w61:dbl[])
        n32 = call-poly <vilib>:"Vector Norm.vi"("Input Vector"=w49) -> ("norm"=w64:dbl)  [unwired: 9 in, 1 out]
        n33 = Divide(x=w49, y=w64) -> (x/y=w46:dbl[])
        n34 = Build Array(w62, w46, w61) -> (w60:T3)
        n35 = call "Matrix Transform Structure.vi"("Matrix Transform"=w60, "Original Structure"="Conventional Unit Cell") -> ("After Transform"=w42:T1)  [unwired: 9 in]
        "Grain 1 Primitive" <- w42
        n36 = Bundle("Z Min"=w59, "Max Grain Width"="Max Grain Width", "Z Min"=w59, "Max Grain Height"="Max Grain Height", "Grain 1 Start"="Grain 1 Start", "Grain 1 Min Length (A)"="Grain 1 Min Length (A)") -> (w40:T4)  [unwired: 1 in]
        n37 = local read "Lattice Parameter"() -> (w38:dbl)
        n38 = Multiply(x=w40, y=w38) -> (x*y=w39:T4)
        n39 = call "Supercell Structure into a Box.vi"("Draw Box"=w39, "Subcrystal"=w42) -> ("Expanded cubic Structure"=w43:T1)  [unwired: 7 in, 2 out]
        "Grain 1" <- w43
        n40 = local read "Grain 1 Object"() -> (w52:refnum<vi>)
        n41 = stacked-sequence {
          tunnel: w43 -> [_]
          frame #0 {
            n42 = property on="Make GB" class="Bool (strict)"("Val(Sgnl)"=TRUE ("Value (Signaling)")) -> ()  [unwired: 2 in, 2 out]
          }
        }
        n43 = Close Reference(reference=w52) -> (error out=w51:errorcluster)  [unwired: 1 in]
        n44 = call <vilib>:"Create Object.vi"("error in (no error)"=w51, "Name"="Base") -> ("Scene:New Object"=w55:refnum<vi>)  [unwired: 9 out]
        n45 = call "Render Structure.vi"("Options"="Options", "Scale"="Scale", "Atomic Structure"=w43, "Base Object"=w55) -> ("Object with atoms"=w50:refnum<vi>)  [unwired: 7 in]
        "Grain 1 Render" <- w50
        n46 = local write "Grain 1 Object"(w50) -> ()
      }
      event "Add Tilt Angle": Value Change {
        n47 = event-data() -> ()  [unwired: 1 in, 5 out]
        n48 = local read "Mutual Viewing Angle"() -> (w67:dbl[])
        n49 = local read "Grain 1 Orientation"() -> (w69:dbl[])
        n50 = call "Make Rotation Matrix.vi"("Rotation Axis"=w67, "Rotation Angle (Degree)"="Add Tilt Angle") -> ("Rotation Matrix"=w70:T3)  [unwired: 9 in]
        n51 = call-poly <vilib>:"A x B.vi"("Matrix A"=w70, "Vector V'"=w69) -> ("V' x A"=w68:dbl[])  [unwired: 1 out]
        n52 = property on="Grain 2 Orientation" class="Arr (strict)"("Val(Sgnl)"=w68) -> ()  [unwired: 2 in, 2 out]
      }
      event "Grain 2 Min Length", "Overlap Region", "Twist Angle", "Translation Vector", "Make Grain 2": Value Change {
        w102 = 0.0 ("Grain 1 Start")
        n53 = event-data() -> ()  [unwired: 1 in, 5 out]
        n54 = local read "Mutual Viewing Angle"() -> (w83:dbl[])
        n55 = local read "Grain 1 Orientation"() -> (w78:dbl[])
        n56 = call "Angle between two vectors.vi"("Vector 2"="Grain 2 Orientation", "Vector 1"=w78) -> ("Angle (Degrees)"=w86:dbl)  [unwired: 7 in, 2 out]
        n57 = call-poly <vilib>:"Vector Norm.vi"("Input Vector"=w83) -> ("norm"=w108:dbl)  [unwired: 9 in, 1 out]
        n58 = call <vilib>:"Cross Product.vi"("B Vector"="Grain 2 Orientation", "A Vector"=w83) -> ("Cross Product"=w103:dbl[])  [unwired: 8 in, 1 out]
        n59 = call-poly <vilib>:"Vector Norm.vi"("Input Vector"="Grain 2 Orientation") -> ("norm"=w106:dbl)  [unwired: 9 in, 1 out]
        n60 = local write "Add Tilt Angle"(w86) -> ()
        n61 = Divide(x=w83, y=w108) -> (x/y=w105:dbl[])
        n62 = Divide(x="Grain 2 Orientation", y=w106) -> (x/y=w104:dbl[])
        n63 = call-poly <vilib>:"Vector Norm.vi"("Input Vector"=w103) -> ("norm"=w107:dbl)  [unwired: 9 in, 1 out]
        n64 = Divide(x=w103, y=w107) -> (x/y=w82:dbl[])
        n65 = Build Array(w105, w82, w104) -> (w79:T3)
        n66 = local read "Conventional Unit Cell"() -> (w75:T1)
        n67 = call-poly <vilib>:"A x B.vi"("Vector"=w78, "A"=w79) -> ("A x Vector"=w77:dbl[])  [unwired: 1 out]
        n68 = local read "Lattice Parameter"() -> (w72:dbl)
        n69 = call "Make Rotation Matrix.vi"("Rotation Axis"=w77, "Rotation Angle (Degree)"="Twist Angle") -> ("Rotation Matrix"=w80:T3)  [unwired: 9 in]
        n70 = call-poly <vilib>:"A x B.vi"("B"=w79, "A"=w80) -> ("A x B"=w88:T3)  [unwired: 1 out]
        n71 = call "Matrix Transform Structure.vi"("Matrix Transform"=w88, "Original Structure"=w75) -> ("After Transform"=w85:T1)  [unwired: 9 in]
        n72 = call "Translate Structure.vi"("Translation Vector (Cartesian)"="Translation Vector", "Atomic Structure"=w85) -> ("Shifted Structure"=w76:T1)  [unwired: 9 in]
        "Grain 2 Primative" <- w76
        n73 = local read "Max Grain Height"() -> (w99:dbl)
        n74 = local read "Max Grain Width"() -> (w87:dbl)
        n75 = Negate(x="Overlap Region") -> (-x=w90:dbl)
        n76 = Bundle("Grain 1 Start"=w102, "Max Grain Width"=w87, "Grain 1 Start"=w102, "Max Grain Height"=w99, w90, "Grain 2 Min Length"="Grain 2 Min Length") -> (w74:T5)  [unwired: 1 in]
        n77 = Multiply(x=w74, y=w72) -> (x*y=w73:T5)
        n78 = call "Supercell Structure into a Box.vi"("Draw Box"=w73, "Subcrystal"=w76) -> ("Expanded cubic Structure"=w95:T1)  [unwired: 7 in, 2 out]
        "Grain 2" <- w95
        n79 = local read "Grain 2 Object"() -> (w93:refnum<vi>)
        n80 = local read "Scale"() -> (w97:dbl)
        n81 = stacked-sequence {
          tunnel: w95 -> [_]
          frame #0 {
            n82 = property on="Make GB" class="Bool (strict)"("Val(Sgnl)"=TRUE ("Value (Signaling)")) -> ()  [unwired: 2 in, 2 out]
          }
        }
        n83 = local read "Options"() -> (w96:cluster{"Border?":bool, "Bonds?":bool})
        n84 = Close Reference(reference=w93) -> (error out=w92:errorcluster)  [unwired: 1 in]
        n85 = call <vilib>:"Create Object.vi"("error in (no error)"=w92, "Name"="Base") -> ("Scene:New Object"=w100:refnum<vi>)  [unwired: 9 out]
        n86 = call "Render Structure.vi"("Options"=w96, "Scale"=w97, "Atomic Structure"=w95, "Base Object"=w100) -> ("Object with atoms"=w94:refnum<vi>)  [unwired: 7 in]
        "Grain 2 Render" <- w94
        n87 = local write "Grain 2 Object"(w94) -> ()
      }
      event "Make GB": Value Change {
        w135 = "," ("string")
        w151 = "," ("string")
        n88 = event-data() -> ()  [unwired: 1 in, 5 out]
        n89 = local read "Grain 1"() -> (w166:T1)
        n90 = Unbundle By Name(w166) -> ("Lattice vector c"=w111:dbl[])
        n91 = local read "Grain 2"() -> (w171:T1)
        n92 = local read "Grain 1 Orientation"() -> (w118:dbl[])
        n93 = local read "Grain 2 Orientation"() -> (w117:dbl[])
        n94 = local read "Translation Vector"() -> (w141:dbl[])
        n95 = local read "Add Tilt Angle"() -> (w147:dbl)
        n96 = local read "Twist Angle"() -> (w116:dbl)
        n97 = Number To Fractional String(number=w147, precision (6)=i16 1) -> (F-format string=w145:string)  [unwired: 2 in]
        n98 = Number To Decimal String(number=w117) -> (decimal integer string=w148:string[])  [unwired: 1 in]
        n99 = Number To Fractional String(number=w141, precision (6)=i16 2) -> (F-format string=w139:string[])  [unwired: 2 in]
        n100 = Number To Decimal String(number=w118) -> (decimal integer string=w149:string[])  [unwired: 1 in]
        n101 = Index Array(array=w149) -> (element #1=w158:string, element #2=w156:string, element #3=w155:string)  [unwired: 3 in]
        n102 = Index Array(array=w148) -> (element #1=w153:string, element #2=w152:string, element #3=w150:string)  [unwired: 3 in]
        n103 = Index Array(array=w139) -> (element #1=w138:string, element #2=w136:string, element #3=w134:string)  [unwired: 3 in]
        n104 = Number To Fractional String(number=w116, precision (6)=i16 1) -> (F-format string=w160:string)  [unwired: 2 in]
        n105 = local read "Options"() -> (w167:cluster{"Border?":bool, "Bonds?":bool})
        n106 = Concatenate Strings("(" ("string"), w138, w135, w136, w135, w134, ")T " ("string")) -> (w132:string)
        n107 = call "Merge Two Structures.vi"("Translation Vector (1 to 2)"=w111, "Atomic Structure 2"=w171, "Atomic Structure 1"=w166) -> ("Atomic Structure of 1 + 2 by T"=w121:T1)  [unwired: 8 in]
        n108 = Concatenate Strings("(" ("string"), w160, ") twist [" ("string"), w158, "," ("string"), w156, w151, w155, "] [" ("string"), w153, w151, w152, w151, w150, "+" ("string"), w145, "tilt] " ("string"), w132, "GB" ("string")) -> (w120:string)
        n109 = Bundle By Name(cluster=w121, "Structure Name"=w120) -> (→"Grain Boundary":T1)
        n110 = local read "Scale"() -> (w168:dbl)
        n111 = local write "Structure Name"(w120) -> ()
        n112 = disable-structure shown="Disabled" {
          disable-tunnel: w118 -> [w180 _]
          disable-tunnel: w117 -> [w179 _]
          disable-tunnel: w116 -> [w178 _]
          disable-tunnel: [w176 _] -> w115
          disable-tunnel: [w175 _] -> w114
          disable-tunnel: [w174 _] -> w113
          disable-tunnel: [w173 _] -> w112
          disable-tunnel: [w172 _] -> w110
          frame Disabled {
            n113 = call "Analyze GB.vi"("Integer Tolerance"=0.1, "Twist Angle (Deg)"=w178, "Grain 2 Orientation"=w179, "Grain 1 Orientation"=w180) -> ("Misorientation Angle"=w173:dbl, "Grain 2 Integers"=w174:dbl[], "Grain 1 Integers"=w175:dbl[], "Suggested Viewing Angle"=w172:dbl[], "Viewable?"=w176:bool)  [unwired: 3 out]
          }
          frame Enabled {
          }
        }
        "Suggested Viewing Angle" <- w110
        "Viewable?" <- w115
        "Grain 1 Integers" <- w114
        "Grain 2 Integers" <- w113
        "Misorientation Angle" <- w112
        n114 = Unbundle By Name(w121) -> ("# of atoms"=→"# of Atoms":i32)
        n115 = local read "Grain Boundary Object"() -> (w164:refnum<vi>)
        n116 = Unbundle By Name(w121) -> ("# of atoms"=w125:i32, "Lattice vector a"=w130:dbl[], "Lattice vector b"=w129:dbl[], "Lattice vector c"=w128:dbl[])
        n117 = call <vilib>:"Cross Product.vi"("B Vector"=w128, "A Vector"=w129) -> ("Cross Product"=w127:dbl[])  [unwired: 8 in, 1 out]
        n118 = Close Reference(reference=w164) -> (error out=w163:errorcluster)  [unwired: 1 in]
        n119 = call-poly <vilib>:"Dot Product.vi"("Y Vector"=w127, "X Vector"=w130) -> ("X * Y"=w126:dbl)  [unwired: 1 out]
        n120 = Divide(x=w125, y=w126) -> (x/y=w124:dbl)
        "Atoms / A³" <- w124
        n121 = call <vilib>:"Create Object.vi"("error in (no error)"=w163, "Name"="Base") -> ("Scene:New Object"=w169:refnum<vi>)  [unwired: 9 out]
        n122 = call "Render Structure.vi"("Options"=w167, "Scale"=w168, "Atomic Structure"=w121, "Base Object"=w169) -> ("Object with atoms"=w165:refnum<vi>)  [unwired: 7 in]
        "Grain Boundary Render" <- w165
        n123 = local write "Grain Boundary Object"(w165) -> ()
        n124 = Divide(x=w124, y=0.0276277) -> (x/y=→"% of Bulk atomic density":dbl)
      }
      event "Crop to Smallest Repeating": Value Change {
        n125 = event-data() -> ()  [unwired: 1 in, 5 out]
        n126 = local read "Grain Boundary"() -> (w192:T1)
        n127 = call "Find Repeating Ortho-Subset in GB.vi"("Presorted?"="Presorted?", "Tolerance (A)"="Tolerance (A)", "Slab Y"="Slab Y", "Slab X"="Slab X", "Grain Boundary"=w192) -> ("Repeating Y Length Scale"=w184:dbl, "Subset Y found?!"=w183:bool, "Repeating X Length Scale"=w186:dbl, "Subset X found?!"=w185:bool)  [unwired: 3 in]
        "Repeating X Length Scale" <- w186
        "Subset for X?" <- w185
        "Repeating Y Length Scale" <- w184
        "Subset for Y?" <- w183
        n128 = case shown="True" w185 {
          tunnel: w192 -> [w206 w211]
          tunnel: [w206 w208] -> w187
          tunnel: w186 -> [_ w207]
          frame False {
          }
          frame True {
            n129 = call "Crop Structure.vi"("Cropping Index"=enum16{"X", "Y", "Z"}."X", "Upper Bound Z"=w207, "Lower bound Z"=0.0, "Input Structure"=w211) -> ("Cropped Structure"=w208:T1)  [unwired: 7 in]
          }
        }
        n130 = case shown="True" w183 {
          tunnel: w187 -> [w200 w205]
          tunnel: w184 -> [_ w203]
          tunnel: [w200 w201] -> w182
          frame False {
          }
          frame True {
            n131 = call "Crop Structure.vi"("Cropping Index"=enum16{"X", "Y", "Z"}."Y", "Upper Bound Z"=w203, "Lower bound Z"=0.0, "Input Structure"=w205) -> ("Cropped Structure"=w201:T1)  [unwired: 7 in]
          }
        }
        n132 = local read "Grain Boundary Object"() -> (w195:refnum<vi>)
        n133 = Unbundle By Name(w182) -> ("# of atoms"=w181:i32)
        n134 = local write "Grain Boundary"(w182) -> ()
        n135 = local read "Scale"() -> (w196:dbl)
        n136 = local read "Options"() -> (w197:cluster{"Border?":bool, "Bonds?":bool})
        n137 = local write "# of Atoms"(w181) -> ()
        n138 = Close Reference(reference=w195) -> (error out=w193:errorcluster)  [unwired: 1 in]
        n139 = call <vilib>:"Create Object.vi"("error in (no error)"=w193, "Name"="Base") -> ("Scene:New Object"=w198:refnum<vi>)  [unwired: 9 out]
        n140 = call "Render Structure.vi"("Options"=w197, "Scale"=w196, "Atomic Structure"=w182, "Base Object"=w198) -> ("Object with atoms"=w194:refnum<vi>)  [unwired: 7 in]
        n141 = local write "Grain Boundary Object"(w194) -> ()
        n142 = local write "Grain Boundary Render"(w194) -> ()
      }
      event "Remove Close Atoms": Value Change {
        n143 = event-data() -> ()  [unwired: 1 in, 5 out]
        n144 = local read "Grain 1 Start"() -> (w214:dbl)
        n145 = local read "Grain 1 Min Length (A)"() -> (w215:dbl)
        n146 = local read "Grain Boundary"() -> (w220:T1)
        n147 = Subtract(x=w215, y=w214) -> (x-y=w213:dbl)
        n148 = call "Remove Close Atoms on GB.vi"("Grain Boundary Location (A)"=w213, "Edge Duplication Range"=3.0, "Minimally Allowable Distance (A)"="Minimally Allowable Distance (A)", "Structure"=w220) -> ("# of Atoms Removed"=→"# of Atoms Removed":i32, "Structure with atoms removed"=w218:T1)  [unwired: 6 in]
        n149 = local read "Grain Boundary Object"() -> (w223:refnum<vi>)
        n150 = local write "Grain Boundary"(w218) -> ()
        n151 = local read "Scale"() -> (w224:dbl)
        n152 = local read "Options"() -> (w225:cluster{"Border?":bool, "Bonds?":bool})
        n153 = Close Reference(reference=w223) -> (error out=w221:errorcluster)  [unwired: 1 in]
        n154 = call <vilib>:"Create Object.vi"("error in (no error)"=w221, "Name"="Base") -> ("Scene:New Object"=w219:refnum<vi>)  [unwired: 9 out]
        n155 = call "Render Structure.vi"("Options"=w225, "Scale"=w224, "Atomic Structure"=w218, "Base Object"=w219) -> ("Object with atoms"=w222:refnum<vi>)  [unwired: 7 in]
        n156 = local write "Grain Boundary Object"(w222) -> ()
        n157 = local write "Grain Boundary Render"(w222) -> ()
      }
      event "Save to POSCAR": Value Change {
        n158 = event-data() -> ()  [unwired: 1 in, 5 out]
        n159 = call "File Dialog"() -> ("selected path"=w230:path)  [unwired: 12 in, 3 out]
        n160 = Build Path(base path=w230, name or relative path="Structure Name") -> (appended path=w228:path)
        n161 = Create Folder(path (use dialog)=w228) -> (created path=w227:path)  [unwired: 2 in, 2 out]
        n162 = stacked-sequence {
          tunnel: "Structure Name" -> [w232 _]
          tunnel: w227 -> [w231 w272]
          frame #0 {
            n163 = local read "Grain Boundary"() -> (w237:T1)
            n164 = Build Path(base path=w231, name or relative path="POSCAR") -> (appended path=w234:path)
            n165 = Bundle By Name(cluster=w237, "Structure Name"=w232) -> (w236:T1)
            n166 = call "Atoms to POSCAR.vi"("Atomic Structure"=w236) -> ("POSCAR File"=w233:string)  [unwired: 10 in]
            n167 = Write to Text File(file (use dialog)=w234, text=w233) -> ()  [unwired: 2 in, 3 out]
          }
          frame #1 {
            w247 = "," ("string")
            w244 = i16 2 ("precision (6)")
            w263 = "," ("string")
            w266 = "," ("string")
            n168 = local read "Grain 1 Orientation"() -> (w256:dbl[])
            n169 = local read "Grain 2 Orientation"() -> (w258:dbl[])
            n170 = local read "Translation Vector"() -> (w245:dbl[])
            n171 = Build Path(base path=w272, name or relative path="README.txt") -> (appended path=w274:path)
            n172 = Number To Fractional String(number=w256, precision (6)=w244) -> (F-format string=w255:string[])  [unwired: 2 in]
            n173 = Number To Fractional String(number=w258, precision (6)=w244) -> (F-format string=w257:string[])  [unwired: 2 in]
            n174 = Number To Fractional String(number=w245, precision (6)=w244) -> (F-format string=w250:string[])  [unwired: 2 in]
            n175 = local read "Overlap Region"() -> (w242:dbl)
            n176 = local read "Add Tilt Angle"() -> (w260:dbl)
            n177 = Index Array(array=w255) -> (element #1=w268:string, element #2=w267:string, element #3=w265:string)  [unwired: 3 in]
            n178 = Index Array(array=w257) -> (element #1=w261:string, element #2=w262:string, element #3=w264:string)  [unwired: 3 in]
            n179 = Index Array(array=w250) -> (element #1=w249:string, element #2=w248:string, element #3=w246:string)  [unwired: 3 in]
            n180 = local read "Grain 1 Start"() -> (w240:dbl)
            n181 = local read "Twist Angle"() -> (w259:dbl)
            n182 = Concatenate Strings(w268, w266, w267, w266, w265) -> (w254:string)
            n183 = Concatenate Strings(w261, w263, w262, w263, w264) -> (w253:string)
            n184 = Number To Fractional String(number=w259) -> (F-format string=w252:string)  [unwired: 3 in]
            n185 = Number To Fractional String(number=w260) -> (F-format string=w251:string)  [unwired: 3 in]
            n186 = Concatenate Strings(w249, w247, w248, w247, w246) -> (w243:string)
            n187 = Number To Fractional String(number=w242) -> (F-format string=w241:string)  [unwired: 3 in]
            n188 = Number To Fractional String(number=w240) -> (F-format string=w239:string)  [unwired: 3 in]
            n189 = Build Array(w254, w253, w252, w251, w243, w241, w239) -> (w238:string[])
            n190 = Build Array(string[] ["Grain 1 Orientation", "Grain 2 Orientation", "Twist Angle (Degree)", "Tilt Angle (Degree)", "Translation (x,y,z)", "Overlap Length (A)", "Grain 1 Start (A)"], w238) -> (w270:string[][])
            n191 = Transpose 2D Array(2D array=w270) -> (transposed array=w269:string[][])
            n192 = call-poly <vilib>:"Write To Spreadsheet File.vi"("2D data"=w269, "file path (dialog if empty)"=w274) -> ()  [unwired: 6 in, 1 out]
          }
        }
      }
      event "Make into GULP": Value Change {
        w285 = "," ("string")
        w282 = i16 2 ("precision (6)")
        w301 = "," ("string")
        w304 = "," ("string")
        n193 = event-data() -> ()  [unwired: 1 in, 5 out]
        n194 = local read "Grain 1 Orientation"() -> (w294:dbl[])
        n195 = local read "Grain 2 Orientation"() -> (w296:dbl[])
        n196 = local read "Translation Vector"() -> (w283:dbl[])
        n197 = Number To Fractional String(number=w294, precision (6)=w282) -> (F-format string=w293:string[])  [unwired: 2 in]
        n198 = Number To Fractional String(number=w296, precision (6)=w282) -> (F-format string=w295:string[])  [unwired: 2 in]
        n199 = Number To Fractional String(number=w283, precision (6)=w282) -> (F-format string=w288:string[])  [unwired: 2 in]
        n200 = local read "Overlap Region"() -> (w280:dbl)
        n201 = local read "Add Tilt Angle"() -> (w298:dbl)
        n202 = Index Array(array=w293) -> (element #1=w306:string, element #2=w305:string, element #3=w303:string)  [unwired: 3 in]
        n203 = Index Array(array=w295) -> (element #1=w299:string, element #2=w300:string, element #3=w302:string)  [unwired: 3 in]
        n204 = Index Array(array=w288) -> (element #1=w287:string, element #2=w286:string, element #3=w284:string)  [unwired: 3 in]
        n205 = local read "Grain 1 Start"() -> (w278:dbl)
        n206 = local read "Twist Angle"() -> (w297:dbl)
        n207 = Concatenate Strings(w306, w304, w305, w304, w303) -> (w292:string)
        n208 = Concatenate Strings(w299, w301, w300, w301, w302) -> (w291:string)
        n209 = Number To Fractional String(number=w297) -> (F-format string=w290:string)  [unwired: 3 in]
        n210 = Number To Fractional String(number=w298) -> (F-format string=w289:string)  [unwired: 3 in]
        n211 = Concatenate Strings(w287, w285, w286, w285, w284) -> (w281:string)
        n212 = Number To Fractional String(number=w280) -> (F-format string=w279:string)  [unwired: 3 in]
        n213 = Number To Fractional String(number=w278) -> (F-format string=w277:string)  [unwired: 3 in]
        n214 = local read "Structure Name"() -> (w312:string)
        n215 = Build Array(w292, w291, w290, w289, w281, w279, w277) -> (w276:string[])
        n216 = Build Array(string[] ["Grain 1 Orientation", "Grain 2 Orientation", "Twist Angle (Degree)", "Tilt Angle (Degree)", "Translation (x,y,z)", "Overlap Length (A)", "Grain 1 Start (A)"], w276) -> (w307:string[][])
        n217 = call <vilib>:"Search and Replace Pattern.vi"("string"=w312, "regular expression (\"\")"="[\\s()\\[\\]]" ("regular expression (\"\")"), "replace string (\"\")"="_" ("replace string (\"\")"), "replace all? (F)"=TRUE) -> ("result string"=w311:string)  [unwired: 1 in, 1 out]
        n218 = Transpose 2D Array(2D array=w307) -> (transposed array=w309:string[][])
        n219 = local read "Grain Boundary"() -> (w322:T1)
        n220 = call "File Dialog2"() -> ("selected path"=w319:path)  [unwired: 12 in, 3 out]
        n221 = Array To Spreadsheet String(array=w309, 3:"%s" ("format string")) -> (spreadsheet string=w275:string)  [unwired: 1 in]
        n222 = Concatenate Strings(w311, ".gin" ("string")) -> (w317:string)
        n223 = Build Path(base path=w319, name or relative path=w317) -> (appended path=w316:path)
        n224 = call "Atoms to GULP File.vi"("Title and Comments"=w275, "Relaxation Type"="Relaxation Type", "Structure"=w322) -> ("GULP File"=w320:string)  [unwired: 8 in]
        n225 = Write to Text File(file (use dialog)=w316, text=w320) -> ()  [unwired: 2 in, 3 out]
      }
      event "Suggest Sizes": Value Change {
        n226 = event-data() -> ()  [unwired: 1 in, 5 out]
        n227 = local read "Mutual Viewing Angle"() -> (w335:dbl[])
        n228 = local read "Grain 1 Orientation"() -> (w346:dbl[])
        n229 = local read "Grain 2 Orientation"() -> (w336:dbl[])
        n230 = local read "Twist Angle"() -> (w337:dbl)
        n231 = local read "Conventional Unit Cell"() -> (w344:T1)
        n232 = call <vilib>:"Cross Product.vi"("B Vector"=w335, "A Vector"=w336) -> ("Cross Product"=w329:dbl[])  [unwired: 8 in, 1 out]
        "Cross Product 2" <- w329
        n233 = call "Make Rotation Matrix.vi"("Rotation Axis"=w336, "Rotation Angle (Degree)"=w337) -> ("Rotation Matrix"=w331:T3)  [unwired: 9 in]
        n234 = call <vilib>:"Cross Product.vi"("B Vector"=w335, "A Vector"=w346) -> ("Cross Product"=w333:dbl[])  [unwired: 8 in, 1 out]
        "Cross Product" <- w333
        n235 = call-poly <vilib>:"A x B.vi"("Vector"=w333, "A"=w331) -> ("A x Vector"=w332:dbl[])  [unwired: 1 out]
        n236 = call-poly <vilib>:"A x B.vi"("Vector"=w329, "A"=w331) -> ("A x Vector"=w330:dbl[])  [unwired: 1 out]
        n237 = call-poly <vilib>:"A x B.vi"("Vector"=w335, "A"=w331) -> ("A x Vector"=w334:dbl[])  [unwired: 1 out]
        n238 = Unbundle By Name(w344) -> ("Lattice vector a"=w343:dbl[], "Lattice vector b"=w342:dbl[], "Lattice vector c"=w341:dbl[])
        n239 = Build Array(w346, w336, w334, w332, w330) -> (w345:dbl[][])
        n240 = for {
          tunnel: w345 -> [w354] mode=indexing
          tunnel: w343 -> [w353]
          tunnel: w342 -> [w352]
          tunnel: w341 -> [w351]
          tunnel: "Tolerance" -> [w350]
          tunnel: [w349] -> w328 mode=indexing
          n241 = call "Find Repeating Length from Direction.vi"("Tolerance"=w350, "Lattice vector c"=w351, "Lattice vector b"=w352, "Lattice vector a"=w353, "Direction"=w354) -> ("Repeating Length (A)"=w349:dbl)  [unwired: 6 in]
        }
        n242 = local read "Lattice Parameter"() -> (w327:dbl)
        n243 = Divide(x=w328, y=w327) -> (x/y=w326:dbl[])
        "x/y" <- w326
        n244 = Index Array(array=w326) -> (element #1=w339:dbl, element #2=w325:dbl, element #3=w338:dbl, element #5=w323:dbl)  [unwired: 5 in, 1 out]
        n245 = property on="Grain 1 Min Length (A)" class="DigNum (strict)"("Val(Sgnl)"=w339) -> (error out=w324:errorcluster)  [unwired: 2 in, 1 out]
        n246 = local write "Grain 2 Min Length"(w325) -> ()
        n247 = local write "Max Grain Height"(w323) -> ()
        n248 = local write "Max Grain Width"(w338) -> ()
        n249 = flat-sequence {
          tunnel: w324 -> [_]
          frame #0 {
            w348 = TRUE ("Value (Signaling)")
            n250 = property on="Make Grain 1" class="Bool (strict)"("Val(Sgnl)"=w348) -> (error out=w347:errorcluster)  [unwired: 2 in, 1 out]
            n251 = property on="Make Grain 2" class="Bool (strict)"(error in=w347, "Val(Sgnl)"=w348) -> ()  [unwired: 1 in, 2 out]
          }
        }
      }
      event "Load G1 VESTA": Value Change {
        n252 = event-data() -> ()  [unwired: 1 in, 5 out]
        n253 = local read "Grain 1 Primitive"() -> (w355:T1)
        n254 = call "Load Structure in VESTA.vi"("Atomic Structure"=w355) -> ()  [unwired: 11 in]
      }
      event "Load G2 VESTA": Value Change {
        n255 = event-data() -> ()  [unwired: 1 in, 5 out]
        n256 = local read "Grain 2 Primative"() -> (w356:T1)
        n257 = call "Load Structure in VESTA.vi"("Atomic Structure"=w356) -> ()  [unwired: 11 in]
      }
      event "Load GB VESTA": Value Change {
        n258 = event-data() -> ()  [unwired: 1 in, 5 out]
        n259 = local read "Grain Boundary"() -> (w357:T1)
        n260 = call "Load Structure in VESTA.vi"("Atomic Structure"=w357) -> ()  [unwired: 11 in]
      }
    }
  }
  n261 = disable-structure shown="Enabled" {
    frame Disabled {
      n262 = local write "Conventional Unit Cell"(T1 {"Structure Name"="CdTe", "Lattice vector a"=[6.615785553057252, 0.0, 0.0], "Lattice vector b"=[0.0, 6.615785553057252, 0.0], "Lattice vector c"=[0.0, 0.0, 6.615785553057252], "Atoms Array"=[{"Atom Name"="Cd", "Positions (Direct)"=[[0.0, 0.0, 0.0], [0.0, 0.5, 0.5], [0.5, 0.0, 0.5], [0.5, 0.5, 0.0]], "Positions (Cartesian)"=[[0.0, 0.0, 0.0], [0.0, 3.307892776528626, 3.307892776528626], [3.307892776528626, 0.0, 3.307892776528626], [3.307892776528626, 3.307892776528626, 0.0]]}, {"Atom Name"="Te", "Positions (Direct)"=[[0.25, 0.25, 0.25], [0.75, 0.75, 0.25], [0.75, 0.25, 0.75], [0.25, 0.75, 0.75]], "Positions (Cartesian)"=[[1.653946388264313, 1.653946388264313, 1.653946388264313], [4.96183916479294, 4.96183916479294, 1.653946388264313], [4.96183916479294, 1.653946388264313, 4.96183916479294], [1.653946388264313, 4.96183916479294, 4.96183916479294]]}], "# of atoms"=8} ("Structure")) -> ()
    }
    frame Enabled {
    }
  }
  n263 = call <vilib>:"Create Object.vi"("Name"="Base") -> ("Scene:New Object"=→"Grain 2 Object":refnum<vi>)  [unwired: 1 in, 9 out]
  n264 = call <vilib>:"Create Object.vi"("Name"="Base") -> ("Scene:New Object"=→"Grain 1 Object":refnum<vi>)  [unwired: 1 in, 9 out]
  n265 = call <vilib>:"Create Object.vi"("Name"="Base") -> ("Scene:New Object"=→"Grain Boundary Object":refnum<vi>)  [unwired: 1 in, 9 out]
  n266 = local read "Conventional Unit Cell"() -> (w2:T1)
  n267 = Unbundle By Name(w2) -> ("Lattice vector a"=w3:dbl[])
  n268 = Square(x=w3) -> (x^2=w4:dbl[])
  n269 = Add Array Elements(numeric array=w4) -> (sum=w5:dbl)
  n270 = Square Root(x=w5) -> (sqrt(x)=→"Lattice Parameter":dbl)
